vi "测试应用程序4.vi"() -> ()   [LabVIEW 2022 SP3]
doc: "本VI是为《我和LabVIEW》一书编写的示例。\n关于本书的介绍请参考网页：\nhttp://ruanqizhen.spaces.live.com/blog/cns!5852D4F797C53FB6!4310.entry"
panel:
  out "数据":dbl
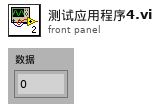
[diagram p1: front panel]
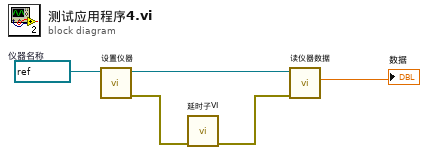
[diagram p0: block diagram]
diagram:
  w3 = refnum<visa-resource-name> "XX仪"  # 仪器名称
  n1 = call "设置仪器.vi"("VISA资源名称"=w3) -> ("error out"=w2:errorcluster, "仪器句柄"=w5:refnum<visa-resource-name>)  [unwired: 1 in, 8 out]
  n2 = call "延时子VI.vi"("error in (no error)"=w2) -> ("error out"=w1:errorcluster)  [unwired: 10 out]
  n3 = call "读仪器数据.vi"("error in (no error)"=w1, "仪器句柄"=w5) -> ("数据"=→"数据":dbl)  [unwired: 9 out]
